vi "Rename Link.vi"(8 "error in (no error)":errorcluster, 9 "New Name":string, 10 "Old Name":string, 11 "Timeout in":refnum<class "Timeout.lvclass">) -> (0 "error out":errorcluster, 3 "Timeout out":refnum<class "Timeout.lvclass">)   [LabVIEW 2015, in "Timeout.lvclass"]
uses:
  Timeout.lvclass
  Timeout.lvclass/Timeout.ctl
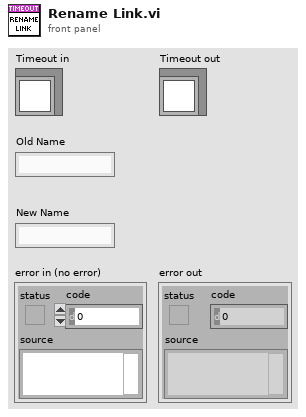
[diagram p1: front panel]
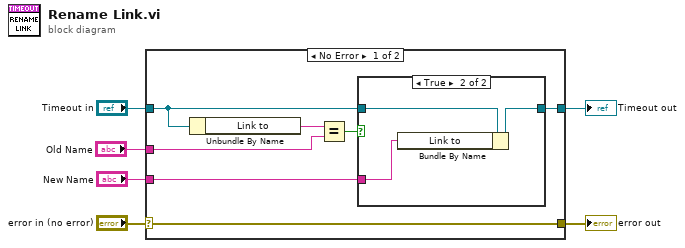
[diagram p0: block diagram]
diagram:
  n1 = case shown="No Error" "error in (no error)" {
    selector: "error in (no error)" -> [w13 w19]
    tunnel: [w13 w19] -> w5
    tunnel: [w12 w18] -> w3
    tunnel: "Timeout in" -> [w10 w18]
    tunnel: "Old Name" -> [w8 _]
    tunnel: "New Name" -> [w7 _]
    frame No Error {
      n2 = Unbundle By Name(w10) -> ("Link to"=w11:string)
      n3 = Equal?(x=w11, y=w8) -> (x = y?=w9:bool)
      n4 = case shown="True" w9 {
        tunnel: w10 -> [w14 w17]
        tunnel: [w14 w16] -> w12
        tunnel: w7 -> [_ w15]
        frame False {
        }
        frame True {
          n5 = Bundle By Name(cluster=w17, "Link to"=w15) -> (w16:refnum<class "Timeout.lvclass">)
        }
      }
    }
    frame Error {
    }
  }
  "error out" <- w5
  "Timeout out" <- w3
